vi "Working Thread.vi"(7 "EngineCSM":string, 10 "SocketName":string, 11 "Sequence":string) -> ()   [LabVIEW 2020, in "CSMStand(Lite).lvlib"]
uses:
  CSMStand(Lite).lvlib
  Typedef/Def-StepComplete Event Data.ctl
  162d78b0-f25f-4e28-9f32-62a227129c30.vi
  3235fbb5-1003-4f8d-8a8e-733f49405df1.vi
  29c90474-5633-4ebd-9475-c7049fde7730.vi
  07558781-58e1-4dd2-b95a-dcbf6018b6a4.vi
  <userlib>/_NEVSTOP/Communicable State Machine(CSM)/AdvanceAPI/CSM - Set Module Attribute.vi
  <userlib>/_NEVSTOP/Communicable State Machine(CSM)/addons/API-String-Arugments-Support/_Support/Data To API String Arguments.vi
  <userlib>/_NEVSTOP/Communicable State Machine(CSM)/AdvanceAPI/CSM - Get Module Attribute.vi
  <userlib>/_NEVSTOP/Communicable State Machine(CSM)/Communicable State Machine.lvlib
  <userlib>/_NEVSTOP/Communicable State Machine(CSM)/_Shared/CSM Shared.lvlib
  <userlib>/_NEVSTOP/Communicable State Machine(CSM)/addons/API-String-Arugments-Support/API String Arguments Support.lvlib
panel:
  in  "Debug Stop":bool
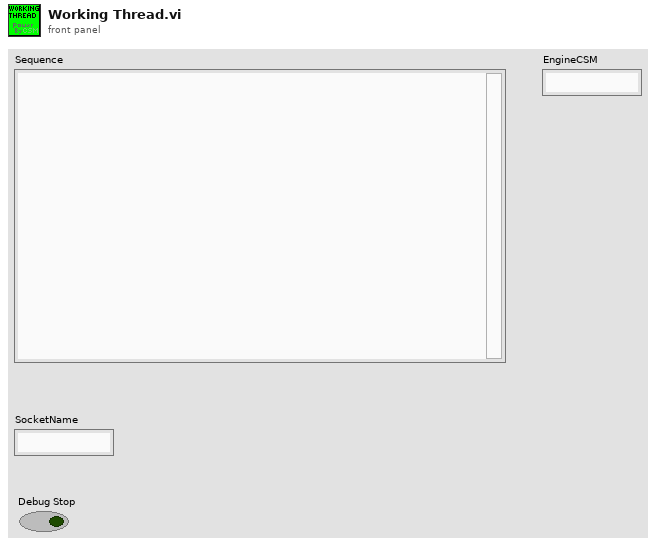
[diagram p1: front panel]
types:
  T1 = typedef "CSMStand(Lite).lvlib/Def-StepComplete Event Data.ctl" = cluster{"index":i32, "Arguments":string, "error":errorcluster}
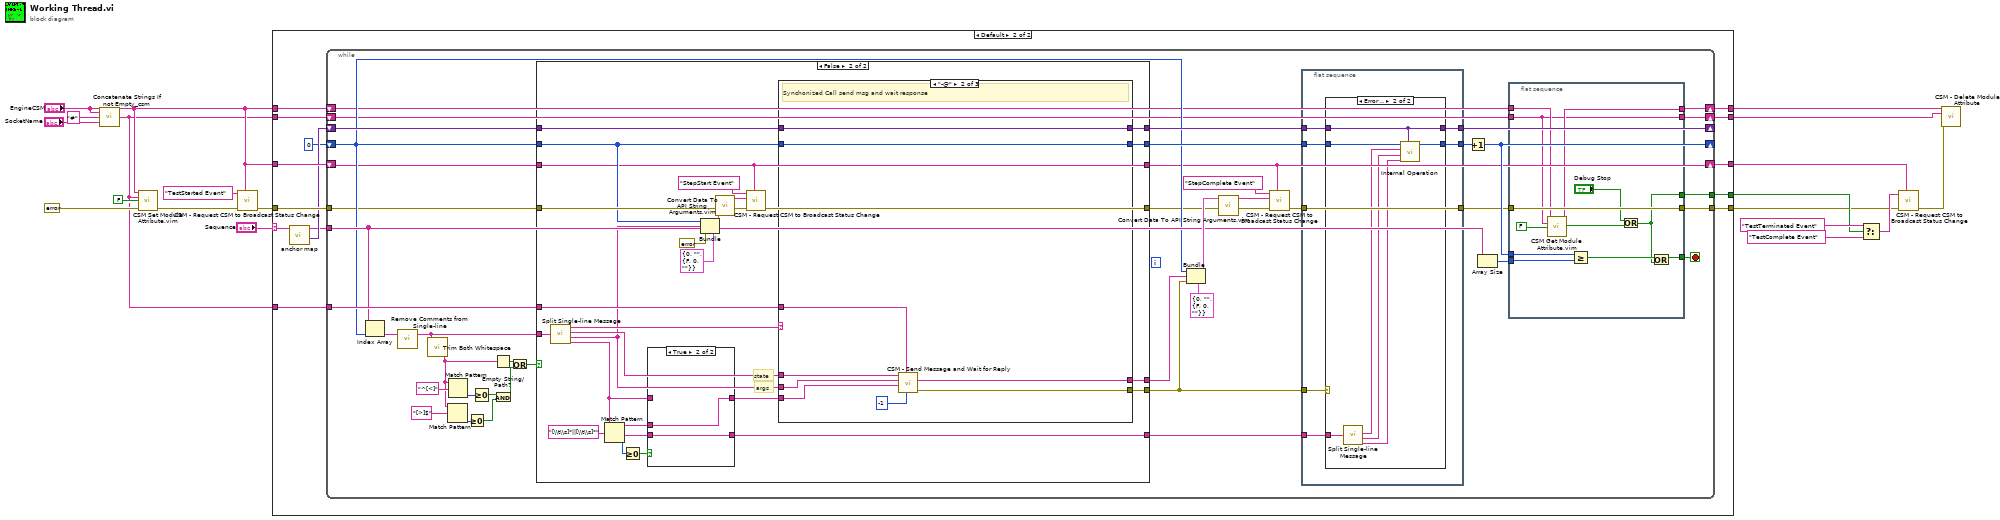
[diagram p0: block diagram]
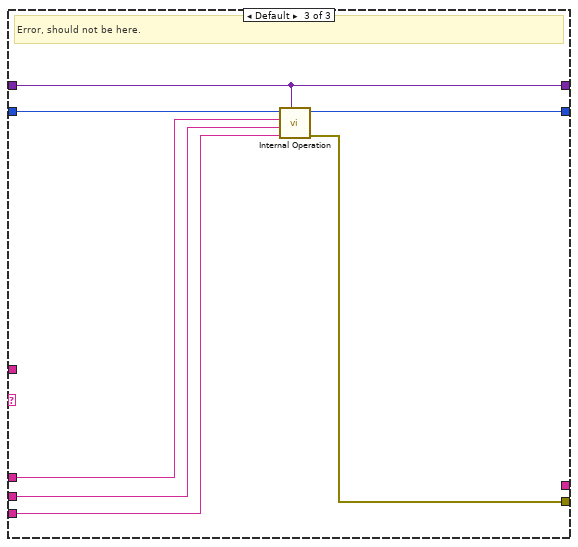
[diagram p7: hidden frame]
diagram:
  n1 = call <userlib>:"Concatenate Strings If not Empty_csm.vi"("String"="SocketName", "seperator(:)"="#", "prefix"="EngineCSM") -> ("result"=w1:string)  [unwired: 2 in]
  n2 = call "CSM Set Module Attribute.vim"("CSM Name"="EngineCSM", "Attribute"=w1, "Value"=FALSE, "Error In"=errorcluster {"status"=FALSE, "code"=0, "source"=""} ("error in (no error)")) -> ("error out"=w5:errorcluster)  [unwired: 8 in, 3 out]
  n3 = call <userlib>:"CSM - Request CSM to Broadcast Status Change.vi"("Module Name"="EngineCSM", "Error In (No Error)"=w5, "Status"="TestStarted Event") -> ("error out"=w18:errorcluster)  [unwired: 8 in]
  n4 = case shown="Default" "Sequence" {
    selector: "Sequence" -> [_ w31]
    tunnel: w18 -> [w22 w37]
    tunnel: "EngineCSM" -> [w23 w36]
    tunnel: [w23 w35] -> w17
    tunnel: [w22 w34] -> w9
    tunnel: w1 -> [_ w33]
    tunnel: "EngineCSM" -> [w21 w28]
    tunnel: [w21 w27] -> w12
    tunnel: [_ w26] -> w10
    tunnel: w1 -> [w20 w25]
    tunnel: [w20 w24] -> w6
    frame "False" {
    }
    frame Default {
      n5 = call "anchor map.vi"("string"=w31) -> ("Archt Map"=w32:variant, "Lines"=w30:string[])  [unwired: 9 in]
      n6 = while {
        tunnel: w37 -> [w43]
        tunnel: [w73] -> w34
        shift-right: [w40] -> w35
        shift-left: w36 -> [w41]
        tunnel: w33 -> [w80]
        tunnel: w30 -> [w70]
        shift-right: [w71] -> _
        shift-left: 0 -> [w47]
        shift-right: [w61] -> _
        shift-left: w32 -> [w68]
        shift-right: [w45] -> w27
        shift-left: w28 -> [w46]
        tunnel: [w44] -> w26
        shift-right: [w38] -> w24
        shift-left: w25 -> [w39]
        stop <- w74 stop-if-true
        n7 = Index Array(array=w70, index=w47) -> (element=w72:string)
        n8 = call <userlib>:"Remove Comments from Single-line.vi"("single-line text"=w72) -> ("single-line text without comments"=w52:string)  [unwired: 2 in]
        n9 = call <userlib>:"Trim Both Whitespace.vi"("String"=w52) -> ("Trimmed String"=w51:string)  [unwired: 1 in]
        n10 = Match Pattern(string=w51, regular expression="[>]$") -> (offset past match=w57:i32)  [unwired: 1 in, 3 out]
        n11 = Match Pattern(string=w51, regular expression="^[<]") -> (offset past match=w58:i32)  [unwired: 1 in, 3 out]
        n12 = Greater Or Equal To 0?(x=w57) -> (x >= 0?=w56:bool)
        n13 = Greater Or Equal To 0?(x=w58) -> (x >= 0?=w55:bool)
        n14 = Empty String/Path?(string/path=w51) -> (empty?=w53:bool)
        n15 = And(x=w55, y=w56) -> (x .and. y?=w54:bool)
        n16 = Or(x=w53, y=w54) -> (x .or. y?=w50:bool)
        n17 = case shown="False" w50 {
          tunnel: w80 -> [_ w138]
          tunnel: [_ w137] -> w64
          tunnel: [_ w136] -> w76
          tunnel: [w112 w135] -> w48
          tunnel: w47 -> [w112 w115]
          tunnel: w68 -> [w111 w134]
          tunnel: [_ w126] -> w63
          tunnel: [w111 w125] -> w62
          tunnel: w52 -> [_ w124]
          tunnel: w43 -> [w110 w120]
          tunnel: [w110 w119] -> w42
          tunnel: w41 -> [w109 w113]
          tunnel: [w109 w113] -> w40
          frame True {
          }
          frame False {
            # "args"
            # "state"
            n18 = call <userlib>:"Split Single-line Message.vi"("single-line text"=w124) -> ("operator"=w140:string, "state"=w139:string, "args"=w114:string, "source/target"=w129:string)  [unwired: 6 in]
            n19 = Match Pattern(string=w129, regular expression="[\\t\\s]*||[\\t\\s]*" ("string")) -> (before substring=w132:string, after substring=w127:string, offset past match=w131:i32)  [unwired: 1 in, 1 out]
            n20 = Greater Or Equal To 0?(x=w131) -> (x >= 0?=w130:bool)
            n21 = case shown="True" w130 {
              tunnel: w132 -> [_ w143]
              tunnel: w129 -> [w141 _]
              tunnel: [w141 w143] -> w128
              tunnel: w127 -> [_ w142]
              tunnel: [_ w142] -> w126
              frame False {
              }
              frame True {
              }
            }
            n22 = Bundle(cluster=T1 {"index"=0, "Arguments"="", "error"={"status"=FALSE, "code"=0, "source"=""}} ("output cluster"), "index"=w115, "Arguments"=w114, "error"=errorcluster {"status"=FALSE, "code"=0, "source"=""}) -> (w117:T1)
            n23 = call "Convert Data To API String Arguments.vim"("error in (no error)"=w120, "data"=w117) -> ("error out"=w122:errorcluster, "String"=w121:string)  [unwired: 6 in]
            n24 = call <userlib>:"CSM - Request CSM to Broadcast Status Change.vi"("Module Name"=w113, "Error In (No Error)"=w122, "Arguments (\"\")"=w121, "Status"="StepStart Event") -> ("error out"=w119:errorcluster)  [unwired: 7 in]
            n25 = case shown="\"-@\"" w140 {
              tunnel: w139 -> [_ w153 w158]
              tunnel: w114 -> [_ w152 w157]
              tunnel: w138 -> [_ w154 _]
              tunnel: w128 -> [_ w151 w156]
              tunnel: [_ w149 w159] -> w137
              tunnel: [_ w148 _] -> w136
              tunnel: [w145 w147 w161] -> w135
              tunnel: w115 -> [w145 w147 w160]
              tunnel: w134 -> [w144 w146 w155]
              tunnel: [w144 w146 w155] -> w125
              frame "->", "->|" {
                # "Async Call and post message to other loop"
              }
              frame "-@" {
                # "Synchonized Call send msg and wait response"
                n26 = call <userlib>:"CSM - Send Message and Wait for Reply.vi"("Response Timeout (-2 Using Global Settings)"=-1 ("Response Timeout(5000ms)"), "Current Module (\"\" to Generate an ID)"=w154, "Target Module"=w151, "Arguments (\"\")"=w152, "State"=w153) -> ("error out"=w149:errorcluster, "Response"=w148:string)  [unwired: 4 in, 1 out]
              }
              frame Default {
                # "Error, should not be here."
                n27 = call "Internal Operation.vi"("Archt Map"=w155, "source/target"=w156, "args"=w157, "state"=w158, "Numeric in"=w160) -> ("error out"=w159:errorcluster, "Numeric out"=w161:i32)  [unwired: 5 in]
              }
            }
          }
        }
        n28 = Bundle(cluster=T1 {"index"=0, "Arguments"="", "error"={"status"=FALSE, "code"=0, "source"=""}} ("output cluster"), "index"=w47, "Arguments"=w76, "error"=w64) -> (w75:T1)
        n29 = call "Convert Data To API String Arguments.vim"("error in (no error)"=w42, "data"=w75) -> ("error out"=w78:errorcluster, "String"=w77:string)  [unwired: 6 in]
        n30 = call <userlib>:"CSM - Request CSM to Broadcast Status Change.vi"("Module Name"=w40, "Error In (No Error)"=w78, "Arguments (\"\")"=w77, "Status"="StepComplete Event") -> ("error out"=w66:errorcluster)  [unwired: 7 in]
        n31 = flat-sequence {
          tunnel: [w85] -> w67
          tunnel: w48 -> [w84]
          tunnel: w66 -> [w87]
          tunnel: [w87] -> w65
          tunnel: w64 -> [w86]
          tunnel: w63 -> [w83]
          tunnel: w62 -> [w82]
          tunnel: [w81] -> w61
          frame #0 {
            n32 = case shown="Error .." w86 {
              tunnel: [w89 w95] -> w85
              tunnel: w84 -> [w89 w96]
              tunnel: w83 -> [_ w94]
              tunnel: w82 -> [w88 w90]
              tunnel: [w88 w90] -> w81
              frame No Error {
              }
              frame Error {
                n33 = call <userlib>:"Split Single-line Message.vi"("single-line text"=w94) -> ("state"=w93:string, "args"=w92:string, "source/target"=w91:string)  [unwired: 6 in, 1 out]
                n34 = call "Internal Operation.vi"("Archt Map"=w90, "source/target"=w91, "args"=w92, "state"=w93, "Numeric in"=w96) -> ("Numeric out"=w95:i32)  [unwired: 5 in, 1 out]
              }
            }
          }
        }
        n35 = Increment(x=w67) -> (x+1=w71:i32)
        n36 = Array Size(array=w70) -> (size(s)=w69:i32)
        n37 = flat-sequence {
          tunnel: [w108] -> w74
          tunnel: [w107] -> w73
          tunnel: w65 -> [w107]
          tunnel: w71 -> [w105]
          tunnel: w69 -> [w104]
          tunnel: w46 -> [w103]
          tunnel: [w102] -> w45
          tunnel: [w100] -> w44
          tunnel: w39 -> [w97]
          tunnel: [w97] -> w38
          frame #0 {
            n38 = call "CSM Get Module Attribute.vim"("CSM Name"=w103, "Attribute"=w97, "Default Value (Empty Variant)"=FALSE) -> ("CSM Name (Dup)"=w102:string, "Value"=w99:bool)  [unwired: 8 in, 3 out]
            n39 = Greater Or Equal?(x=w105, y=w104) -> (x >= y?=w106:bool)
            n40 = Or(x="Debug Stop", y=w99) -> (x .or. y?=w100:bool)
            n41 = Or(x=w106, y=w100) -> (x .or. y?=w108:bool)
          }
        }
      }
    }
  }
  n42 = Select(t="TestTerminated Event" ("Status"), s=w10, f="TestComplete Event" ("Status")) -> (s? t:f=w16:string)
  n43 = call <userlib>:"CSM - Request CSM to Broadcast Status Change.vi"("Module Name"=w17, "Error In (No Error)"=w9, "Status"=w16) -> ("error out"=w11:errorcluster)  [unwired: 8 in]
  n44 = call <userlib>:"CSM - Delete Module Attribute.vi"("CSM Name"=w12, "Attribute"=w6, "Error In"=w11) -> ()  [unwired: 9 in, 4 out]
